vi "Error 5102 - DTACQ unit replied with an error--const.vi"() -> (0 "error out":errorcluster)   [LabVIEW 2017, in "Communications Library.lvlib"]
doc: "Error 5102\n\nError sending a message to the DTACQ device. DTACQ device replied with the word ERROR."
uses:
  Communications Library.lvlib
  <vilib>/Utility/error.llb/Error Cluster From Error Code.vi
  <vilib>/ErrorRing/Error Ring.xnode
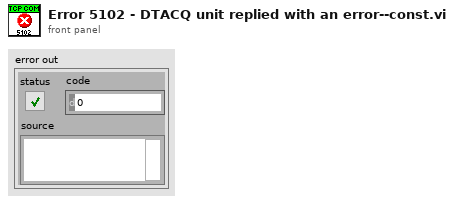
[diagram p1: front panel]
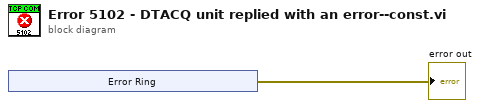
[diagram p0: block diagram]
diagram:
  n1 = xnode "Error Ring"() -> ("error out"=→"error out":errorcluster)
